vi "Set Package.vi"(7 "LabVIEW Web Service Request":refnum<class "Web Request.lvclass">) -> ()   [LabVIEW 2016]
uses:
  <vilib>/wsapi/Web Request.lvclass
  <vilib>/wsapi/class/subVIs/Write Single Session Variable.vi
  WSsupport.lvlib
  ServerErrors/ServerErrors.lvlib
panel:
  # "Use the Web Service Request input terminal to call the VIs on the Web Services palette. Do not remove it from the connector pane unless you don't need access to the palette."
  # "Each additional control wired to the connector pane will be available as an input in the URL. To include an indicator in terminal-mode output (the default setting), it must also be wired to the connector pane."
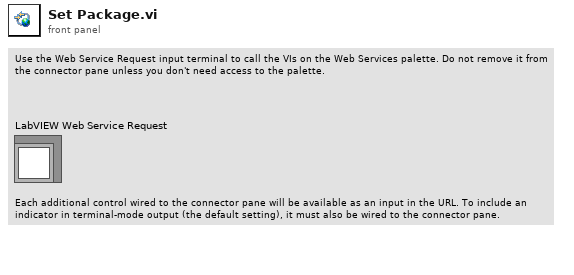
[diagram p1: front panel]
types:
  T1 = typedef "ServerErrors.lvlib/Error Message--cluster.ctl" = cluster{"HTTP Code":i32, "JSON Response":cluster{"error":string, "reason":string}}
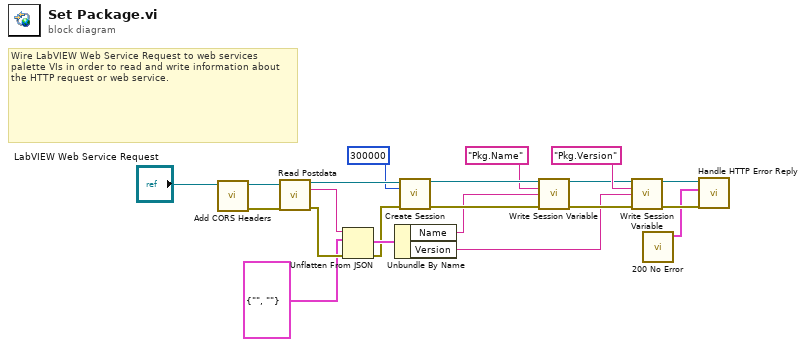
[diagram p0: block diagram]
diagram:
  # "Wire LabVIEW Web Service Request to web services palette VIs in order to read and write information about the HTTP request or web service."
  n1 = call "Add CORS Headers.vi"("LabVIEW Web Service Request"="LabVIEW Web Service Request") -> ("error out"=w19:errorcluster, "LabVIEW Web Service Request out"=w20:refnum<class "Web Request.lvclass">)  [unwired: 9 in]
  n2 = call <vilib>:"Read Postdata.vi"("LabVIEW Web Service Request"=w20, "error in (no error)"=w19) -> ("LabVIEW Web Service Request out"=w14:refnum<class "Web Request.lvclass">, "postdata"=w17:string, "error out"=w18:errorcluster)  [unwired: 11 in]
  n3 = Unflatten From JSON(JSON string=w17, type and defaults=cluster{"Name":string, "Version":string} {"Name"="", "Version"=""}, error in (no error)=w18) -> (value=w15:cluster{"Name":string, "Version":string}, error out=w13:errorcluster)  [unwired: 4 in]
  n4 = Unbundle By Name(w15) -> ("Name"=w8:string, "Version"=w4:string)
  n5 = call <vilib>:"Create Session.vi"("LabVIEW Web Service Request"=w14, "timeout (60000 msec)"=u32 300000, "error in (no error)"=w13) -> ("LabVIEW Web Service Request out"=w11:refnum<class "Web Request.lvclass">, "error out"=w10:errorcluster)  [unwired: 10 in, 1 out]
  n6 = call-poly <vilib>:"Write Session Variable.vi"("LabVIEW Web Service Request"=w11, "key"="Pkg.Name", "value"=w8, "error in (no error)"=w10) -> ("LabVIEW Web Service Request out"=w6:refnum<class "Web Request.lvclass">, "error out"=w5:errorcluster)  [unwired: 8 in, 2 out]
  n7 = call-poly <vilib>:"Write Session Variable.vi"("LabVIEW Web Service Request"=w6, "key"="Pkg.Version", "value"=w4, "error in (no error)"=w5) -> ("LabVIEW Web Service Request out"=w3:refnum<class "Web Request.lvclass">, "error out"=w2:errorcluster)  [unwired: 8 in, 2 out]
  n8 = call "200 No Error.vi"() -> ("no error"=w1:T1)  [unwired: 11 in]
  n9 = call "Handle HTTP Error Reply.vi"("error in (no error)"=w2, "HTTP Status Code"=w1, "Web Request in"=w3) -> ()  [unwired: 8 in, 1 out]
